vi "From Serial Form.vi"(6 "Serial Version":T1, 10 "Deserializer in":refnum<class "Deserializer.lvclass">, 11 "Single in":refnum<class "Single.lvclass">) -> (0 "error out":errorcluster, 2 "Deserializer out":refnum<class "Deserializer.lvclass">, 3 "Single out":refnum<class "Single.lvclass">)   [LabVIEW 2014, in "Base Data Class.lvlib" / "Single.lvclass"]
uses:
  Single.lvclass
  <vilib>/NI/AQ Character Lineator/Deserializer/Deserializer.lvclass
  <vilib>/NI/AQ Character Lineator/Serialization Common/Serial Version.ctl
  Single.lvclass/Single.ctl
  <vilib>/NI/AQ Character Lineator/Serializable/Remove Single.vi
  Data.lvclass
  <vilib>/NI/AQ Character Lineator/Serializable/Serializable.lvclass
  <vilib>/NI/AQ Character Lineator/Serialization Common/Serialization Common.lvlib
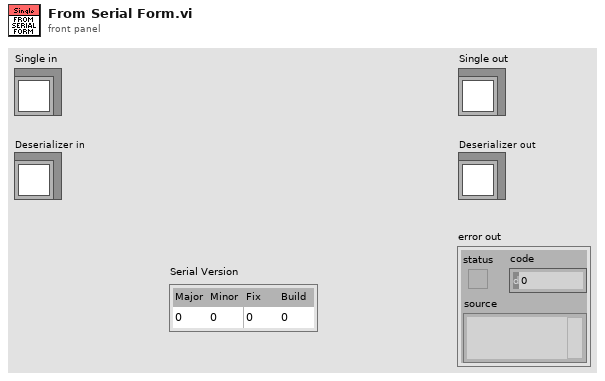
[diagram p1: front panel]
types:
  T1 = typedef "Serialization Common.lvlib/Serial Version.ctl" = cluster{"Major":u16, "Minor":u16, "Fix":u16, "Build":u16}
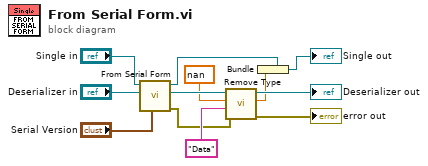
[diagram p0: block diagram]
diagram:
  n1 = call-parent "From Serial Form.vi"("Serial Version"="Serial Version", "Deserializer in"="Deserializer in", "Data in"="Single in") -> ("error out"=w2:errorcluster, "Deserializer out"=w7:refnum<class "Deserializer.lvclass">, "Data out"=w4:refnum<class "Single.lvclass">)  [unwired: 6 in]
  n2 = call-poly <vilib>:"Remove Type.vi"("error in (no error)"=w2, "Name"="Data", "Default Value"=sgl nan, "Deserializer in"=w7) -> ("error out"=→"error out":errorcluster, "Numeric"=w5:sgl, "Deserializer out"=→"Deserializer out":refnum<class "Deserializer.lvclass">)  [unwired: 4 in, 1 out]
  n3 = Bundle(cluster=w4, w5) -> (→"Single out":refnum<class "Single.lvclass">)
